vi "Date pentru predictia hipertensiunii arteriale.vi"() -> ()   [LabVIEW 2024]
panel:
  out "appended array":dbl[][](array[numeric])
  in  "nr minim bauturi alcoolice/saptamana":dbl
  in  "nr maxim bauturi alcoolice/saptamana":dbl
  in  "ore minime de activitati fizice/saptamana":dbl
  in  "ore maxime de activitati fizice/saptamana":dbl
  in  "glicemie minima":dbl
  in  "glicemie maxima":dbl
  in  "colesterol minim":dbl
  in  "colesterol maxim":dbl
  in  "IMC minim":dbl
  in  "IMC maxim":dbl
  in  "varsta minima":dbl
  in  "varsta maxima":dbl
  in  "val esantion":i32
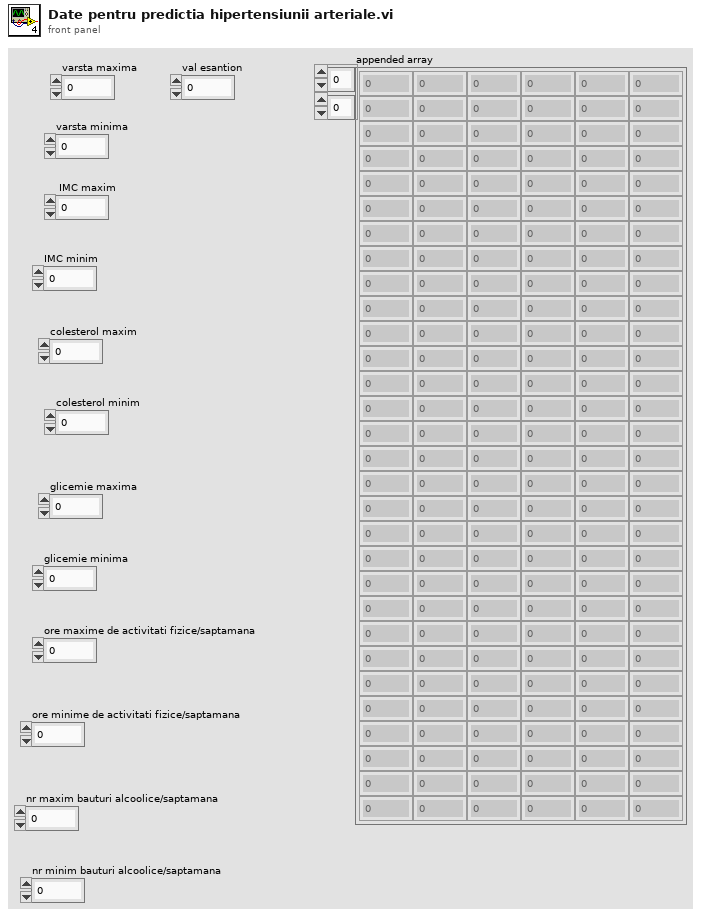
[diagram p1: front panel]
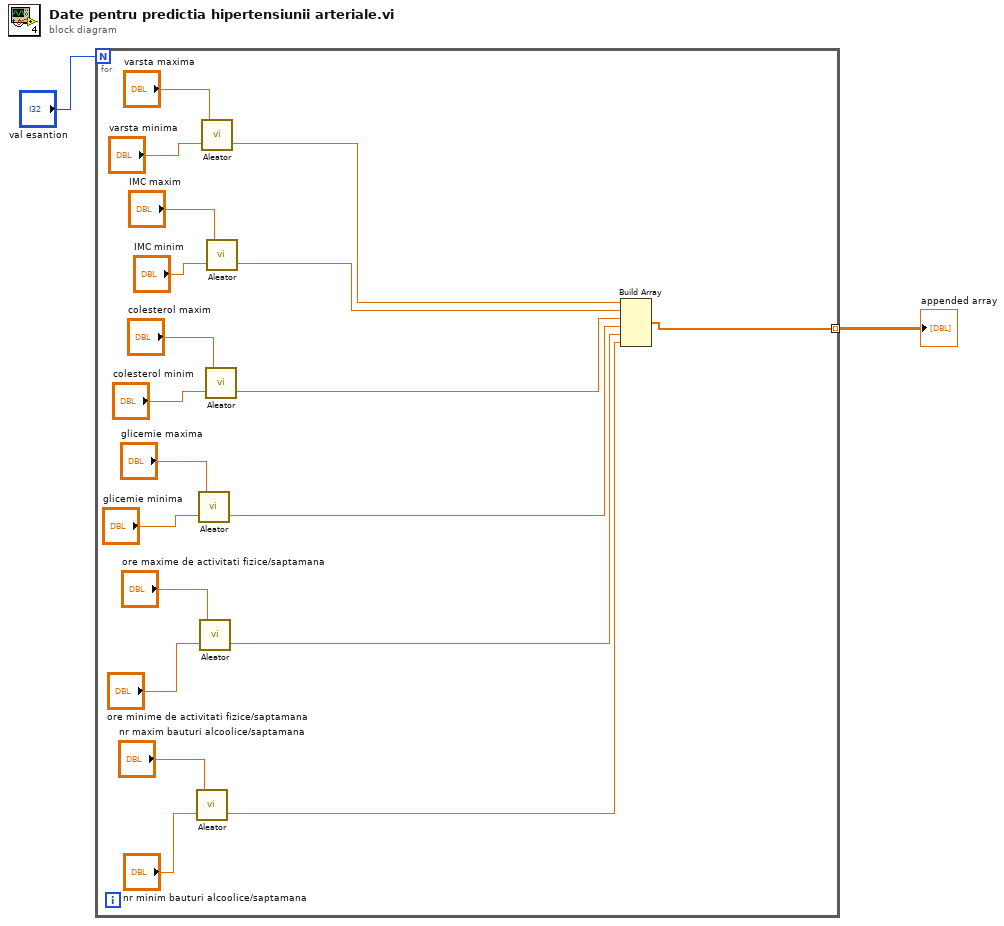
[diagram p0: block diagram]
diagram:
  n1 = for {
    N: "val esantion" -> [_]
    tunnel: [w3] -> w1 mode=indexing
    n2 = call "Aleator.vi"("minim"="nr minim bauturi alcoolice/saptamana", "maxim"="nr maxim bauturi alcoolice/saptamana") -> ("x val aleatoare"=w4:dbl)  [unwired: 1 in]
    n3 = call "Aleator.vi"("minim"="glicemie minima", "maxim"="glicemie maxima") -> ("x val aleatoare"=w6:dbl)  [unwired: 1 in]
    n4 = call "Aleator.vi"("minim"="ore minime de activitati fizice/saptamana", "maxim"="ore maxime de activitati fizice/saptamana") -> ("x val aleatoare"=w5:dbl)  [unwired: 1 in]
    n5 = call "Aleator.vi"("minim"="varsta minima", "maxim"="varsta maxima") -> ("x val aleatoare"=w9:dbl)  [unwired: 1 in]
    n6 = call "Aleator.vi"("minim"="colesterol minim", "maxim"="colesterol maxim") -> ("x val aleatoare"=w7:dbl)  [unwired: 1 in]
    n7 = call "Aleator.vi"("minim"="IMC minim", "maxim"="IMC maxim") -> ("x val aleatoare"=w8:dbl)  [unwired: 1 in]
    n8 = Build Array(w9, w8, w7, w6, w5, w4) -> (w3:dbl[])
  }
  "appended array" <- w1
